vi "Test DO Interconnected Lines.vi"() -> ()   [LabVIEW 2013]
uses:
  SLL DAQ Engine/Software/Source Code/Sub VIs/DAQ Engine/Controls/SLL DE DO Global Options.ctl
  SLL DAQ Engine/Software/Source Code/Sub VIs/DAQ Engine/Controls/SLL DE List of Digital Outputs.ctl
panel:
  in  "Error In":errorcluster
  out "error out":errorcluster
  out "Digital Array Status":bool[](array[boolean])
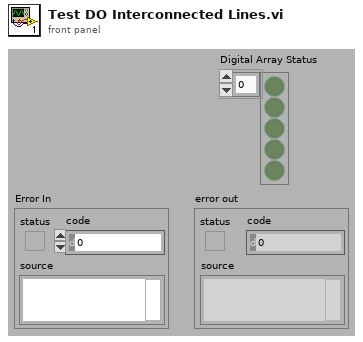
[diagram p1: front panel]
types:
  T1 = typedef "SLL DE List of Digital Outputs.ctl" = enum16{"STATION1_START TEST", "STATION1_STOP TEST", "STATION1_LIGHT1", "STATION1_LIGHT2", "STATION1_LIGHT3", "STATION1_SELECT_TEST", "STATION2_START TEST", "STATION2_STOP TEST", "STATION2_LIGHT1", "STATION2_LIGHT2", "STATION2_LIGHT3", "STATION2_SELECT_TEST", "STATION3_START TEST", "STATION3_STOP TEST", "STATION3_LIGHT1", "STATION3_LIGHT2", "STATION3_LIGHT3", "STATION3_SELECT_TEST", "STATION4_START TEST", "STATION4_STOP TEST", "STATION4_LIGHT1", "STATION4_LIGHT2", "STATION4_LIGHT3", "STATION4_SELECT_TEST"}
  T2 = typedef "SLL DE DO Global Options.ctl" = enum16{"Init", "Write Line", "Write Array", "Write Full Status", "Read Line", "Read Array", "Read Full Status", "Restart DO", "Send to Safe Mode", "Stop DO"}
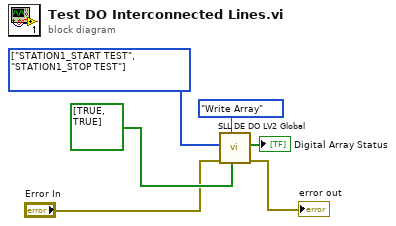
[diagram p0: block diagram]
diagram:
  w5 = T1[] [enum."STATION1_START TEST", enum."STATION1_STOP TEST"] items=["STATION1_START TEST", "STATION1_STOP TEST", "STATION1_LIGHT1", "STATION1_LIGHT2", "STATION1_LIGHT3", "STATION1_SELECT_TEST", "STATION2_START TEST", "STATION2_STOP TEST", "STATION2_LIGHT1", "STATION2_LIGHT2", "STATION2_LIGHT3", "STATION2_SELECT_TEST", "STATION3_START TEST", "STATION3_STOP TEST", "STATION3_LIGHT1", "STATION3_LIGHT2", "STATION3_LIGHT3", "STATION3_SELECT_TEST", "STATION4_START TEST", "STATION4_STOP TEST", "STATION4_LIGHT1", "STATION4_LIGHT2", "STATION4_LIGHT3", "STATION4_SELECT_TEST"] ("DO Channel Name Array")
  n1 = call "SLL DE DO LV2 Global.vi"("DO State Array"=bool[] [TRUE, TRUE], "DO Option"=SLL_DE_DO_Global_Options."Write Array", "Error In"="Error In", "DO Channel Name Array"=w5) -> ("error out"=→"error out":errorcluster, "Digital Array Status"=→"Digital Array Status":bool[])  [unwired: 4 in, 2 out]
